vi "RadiusOfCircleThreePoints.vi"(11 "Points":cluster{"X":dbl, "Y":dbl}[](array[cluster])) -> (3 "R":dbl)   [LabVIEW 2018]
doc: "Find the radius of a circle defined by three points"
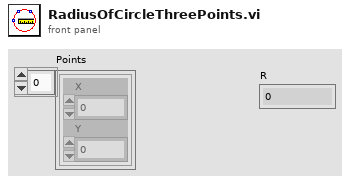
[diagram p1: front panel]
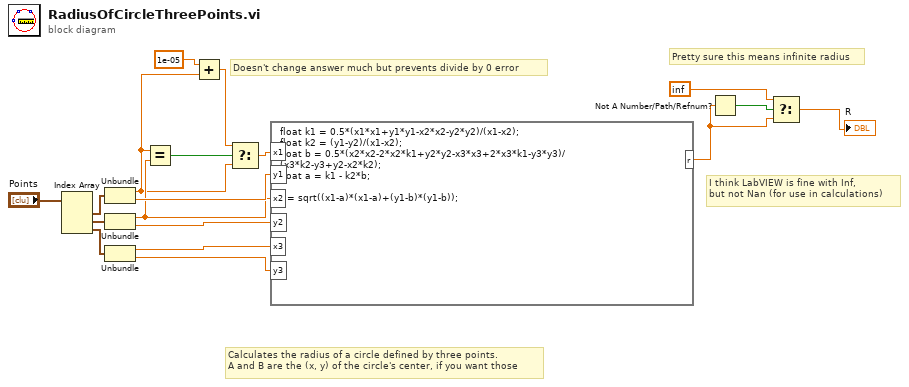
[diagram p0: block diagram]
diagram:
  # "Pretty sure this means infinite radius"
  # "Calculates the radius of a circle defined by three points.\nA and B are the (x, y) of the circle's center, if you want those"
  # "I think LabVIEW is fine with Inf,\nbut not Nan (for use in calculations)"
  # "Doesn't change answer much but prevents divide by 0 error"
  n1 = Index Array(array="Points") -> (element #1=w7:cluster{"X":dbl, "Y":dbl}, element #2=w6:cluster{"X":dbl, "Y":dbl}, element #3=w5:cluster{"X":dbl, "Y":dbl})  [unwired: 3 in]
  n2 = Unbundle(w7) -> ("X"=w11:dbl, "Y"=w18:dbl)
  n3 = Unbundle(w6) -> ("X"=w14:dbl, "Y"=w17:dbl)
  n4 = Unbundle(w5) -> ("X"=w16:dbl, "Y"=w15:dbl)
  n5 = Equal?(x=w11, y=w14) -> (x = y?=w13:bool)
  n6 = Add(x=1e-05, y=w11) -> (x+y=w9:dbl)
  n7 = Select(t=w9, s=w13, f=w11) -> (s? t:f=w12:dbl)
  n8 = formula code="float k1 = 0.5*(x1*x1+y1*y1-x2*x2-y2*y2)/(x1-x2);\nfloat k2 = (y1-y2)/(x1-x2);\nfloat b = 0.5*(x2*x2-2*x2*k1+y2*y2-x3*x3+2*x3*k1-y3*y3)/\n(x3*k2-y3+y2-x2*k2);\nfloat a = k1 - k2*b;\n\nr = sqrt((x1-a)*(x1-a)+(y1-b)*(y1-b));"("x1"=w12, "y1"=w18, "x2"=w14, "y2"=w17, "x3"=w16, "y3"=w15) -> ("r"=w3:dbl)
  n9 = Not A Number/Path/Refnum?(number/path/refnum=w3) -> (NaN/Path/Refnum?=w4:bool)
  n10 = Select(t=inf, s=w4, f=w3) -> (s? t:f=→"R":dbl)
